vi "espectroscopia.vi"() -> ()   [LabVIEW 2016]
uses:
  indicador.ctl
  <vilib>/Utility/file.llb/Write Delimited Spreadsheet (DBL).vi
panel:
  in  "Ref. Mult":dbl
  in  "Ref. LockIn":dbl
  in  "movil":enum16{"acton", "spex"}(ring)
  in  "fijo":enum16{"acton", "spex"}(ring)
  out "medicion":T1
  in  "tipo":bool
  in  "OK Button":bool
  in  "Tab Control":enum32{"medir", "configurar"}(tab)
  out "Lamda Fija":dbl
  in  "Num.Lecturas":i32
  in  "Monocromador movil":cluster{"inicio":dbl, "fin":dbl, "paso":dbl}
  in  "Monocromador fijo":cluster{"Pos.":dbl}
  out "R 2":dbl
  out "DR 2":dbl
  out "DR/R 2":dbl
  out "Lamda":dbl
  in  "file path (use dialog)":path
  in  "spex":bool
  in  "acton":bool
  out "Long Acton":dbl
  in  "longitud Acton":dbl
  out "Longitud  de onda":dbl
  in  "longitud Spex":dbl
  in  "Detener":bool
  out "DR/R":cluster{dbl[], dbl[]}(graph)
  out "R":cluster{dbl[], dbl[]}(graph)
  out "DR":cluster{dbl[], dbl[]}(graph)
  # "PRE"
  # "PR"
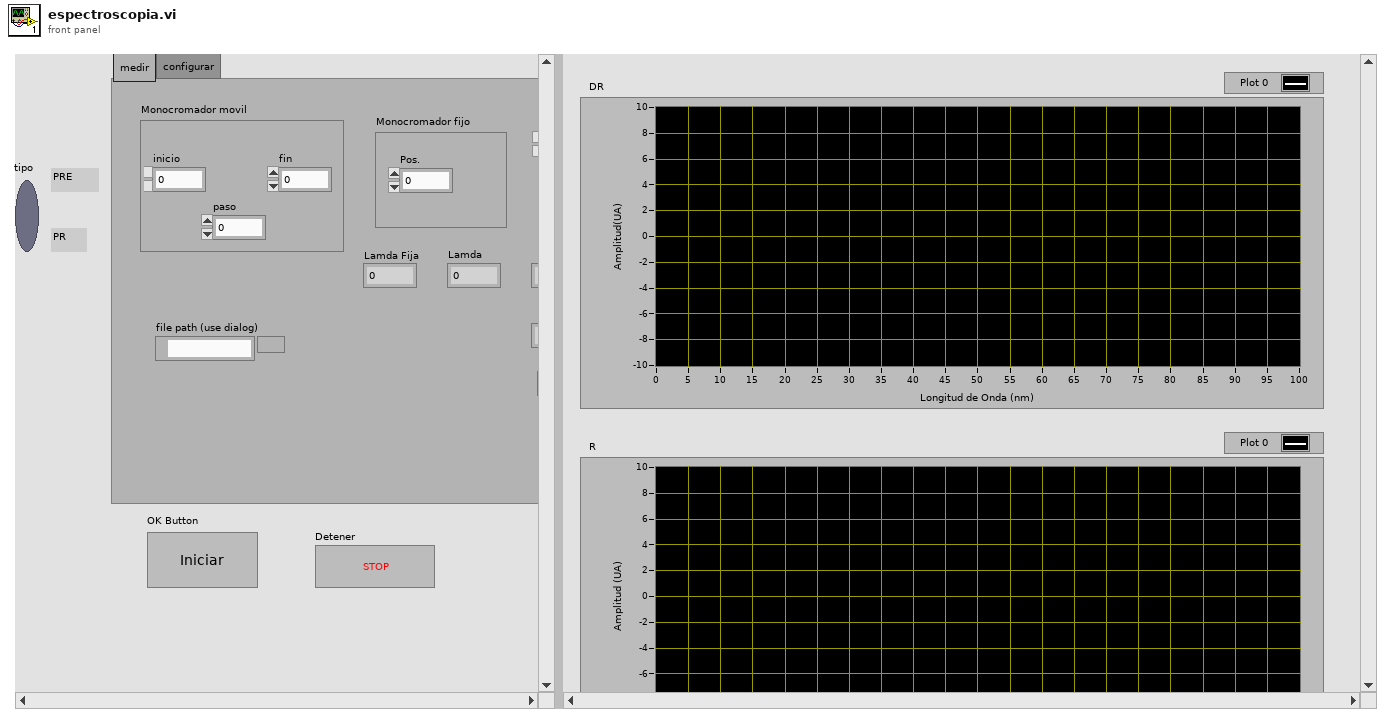
[diagram p1: front panel]
types:
  T1 = typedef "indicador.ctl" = bool
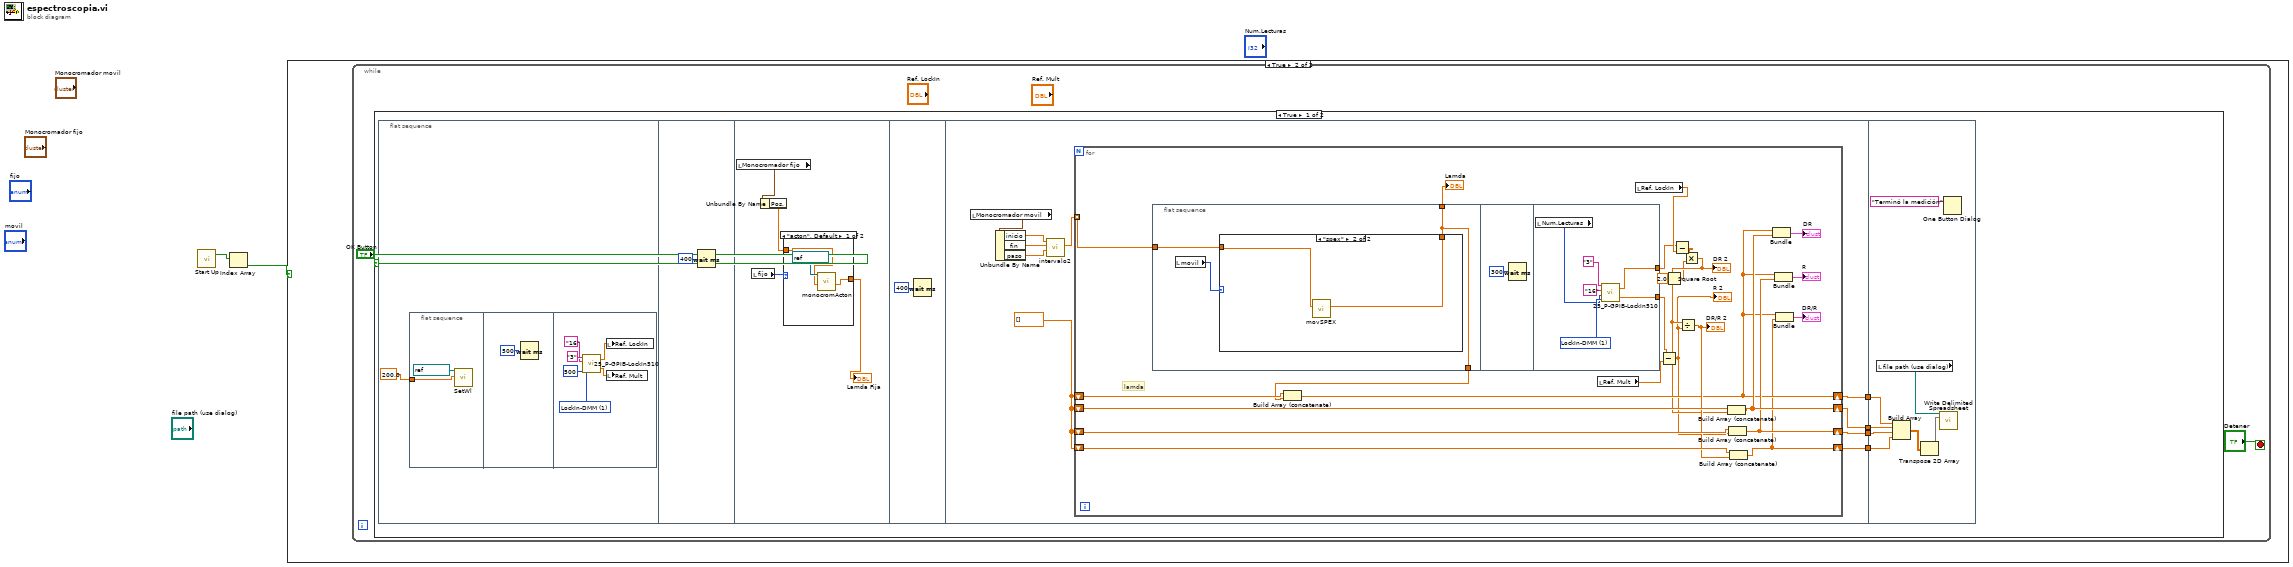
[diagram p0: block diagram]
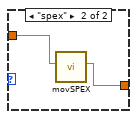
[diagram p3: hidden frame]
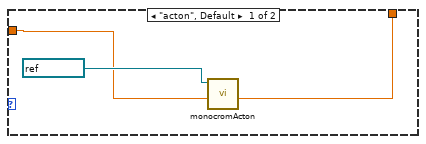
[diagram p4: hidden frame]
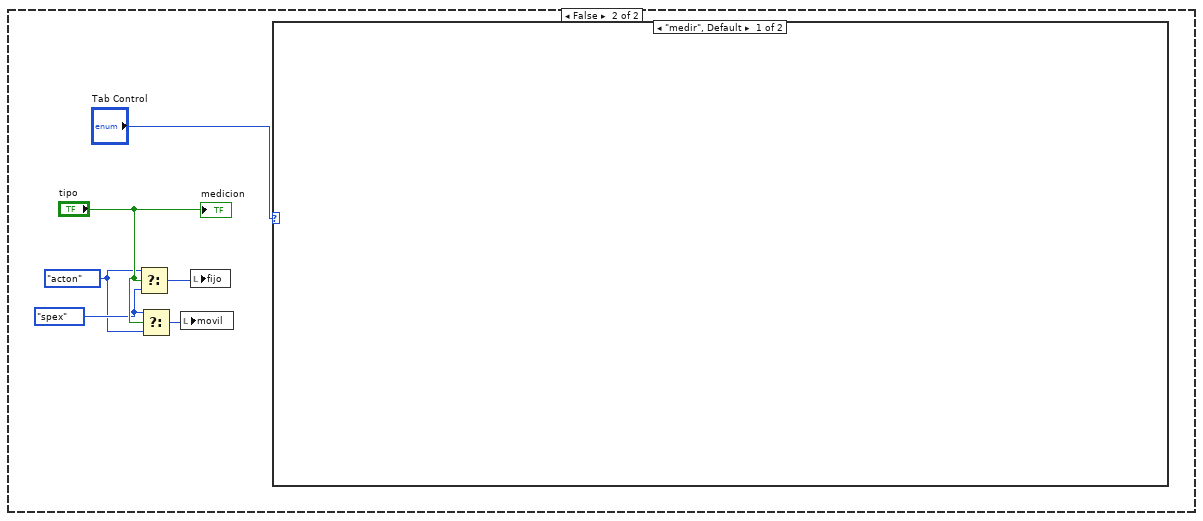
[diagram p5: hidden frame]
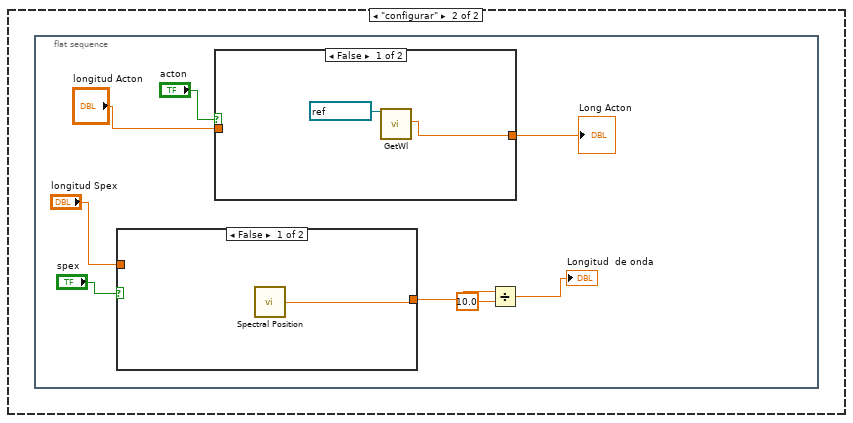
[diagram p6: hidden frame]
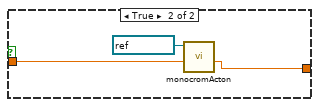
[diagram p7: hidden frame]
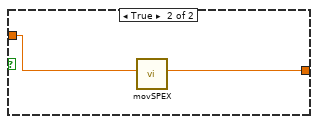
[diagram p8: hidden frame]
diagram:
  n1 = call "Start Up.VI"() -> ("Error List"=w2:bool[])  [unwired: 1 in, 1 out]
  n2 = Index Array(array=w2) -> (element=w1:bool)  [unwired: 1 in]
  n3 = case shown="True" w1 {
    frame False {
    }
    frame True {
      n4 = while {
        stop <- "Detener" stop-if-true
        n5 = case shown="True" "OK Button" {
          frame True {
            n6 = flat-sequence {
              tunnel: [w33] -> w8
              tunnel: [w32] -> w7
              tunnel: [w31] -> w6
              tunnel: [w30] -> w5
              tunnel: w8 -> [w84]
              tunnel: w7 -> [w83]
              tunnel: w6 -> [w82]
              tunnel: w5 -> [w81]
              frame #0 {
                n7 = flat-sequence {
                  tunnel: 200.0 -> [w10]
                  frame #0 {
                    n8 = call "SetWl.vi"("VISA resource name"=refnum<visa-resource-name> "COM5", "Wavelength (nm)"=w10) -> ()  [unwired: 16 in, 2 out]
                  }
                  frame #1 {
                    n9 = Wait (ms)(milliseconds to wait=u32 500) -> ()  [unwired: 1 out]
                  }
                  frame #2 {
                    w13 = u16 1 items=["LockIn", "LockIn-DMM"] ("Tipo")
                    n10 = call "25_P-GPIB-LockIn510.vi"("Tipo"=w13, "Lecturas"=500, "P-DMM"="16", "P-LockIn"="3") -> ("DMM"=w16:dbl, "LockIn"=w15:dbl)
                    n11 = local write "Ref. LockIn"(w15) -> ()
                    n12 = local write "Ref. Mult"(w16) -> ()
                  }
                }
              }
              frame #1 {
                n13 = Wait (ms)(milliseconds to wait=u32 400) -> ()  [unwired: 1 out]
              }
              frame #2 {
                n14 = local read "Monocromador fijo"() -> (w22:cluster{"Pos.":dbl})
                n15 = local read "fijo"() -> (w23:enum16{"acton", "spex"})
                n16 = Unbundle By Name(w22) -> ("Pos."=w21:dbl)
                n17 = case shown="\"acton\", Default" w23 {
                  tunnel: w21 -> [w25 w28]
                  tunnel: [w24 w27] -> w20
                  frame "acton", Default {
                    n18 = call "monocromActon.vi"("Lamda"=w25, "VISA resource name"=refnum<visa-resource-name> "COM3") -> ("Sal:Lamda"=w24:dbl)  [unwired: 9 in]
                  }
                  frame "spex" {
                    n19 = call "movSPEX.vi"("longitud de onda"=w28) -> ("Lamda"=w27:dbl)  [unwired: 10 in]
                  }
                }
                "Lamda Fija" <- w20
              }
              frame #3 {
                n20 = Wait (ms)(milliseconds to wait=u32 400) -> ()  [unwired: 1 out]
              }
              frame #4 {
                w34 = dbl[] []
                n21 = local read "Monocromador movil"() -> (w39:cluster{"inicio":dbl, "fin":dbl, "paso":dbl})
                n22 = Unbundle By Name(w39) -> ("inicio"=w38:dbl, "fin"=w37:dbl, "paso"=w36:dbl)
                n23 = call "intervalo2.vi"("incremento"=w36, "fin"=w37, "inicio"=w38) -> ("Array"=w35:dbl[])  [unwired: 8 in]
                n24 = for {
                  tunnel: w35 -> [w63] mode=indexing
                  shift-right: [w54] -> w32
                  shift-left: w34 -> [w59]
                  shift-right: [w52] -> w31
                  shift-left: w34 -> [w58]
                  shift-right: [w50] -> w30
                  shift-left: w34 -> [w57]
                  shift-right: [w51] -> w33
                  shift-left: w34 -> [w61]
                  # "lamda"
                  n25 = flat-sequence {
                    tunnel: w63 -> [w65]
                    tunnel: [w64] -> w62
                    tunnel: [w64] -> w60
                    tunnel: [w74] -> w45
                    tunnel: [w73] -> w41
                    frame #0 {
                      n26 = local read "movil"() -> (w66:enum16{"acton", "spex"})
                      n27 = case shown="\"spex\"" w66 {
                        tunnel: w65 -> [w68 w71]
                        tunnel: [w67 w70] -> w64
                        frame "acton", Default {
                          n28 = call "monocromActon.vi"("Lamda"=w68, "VISA resource name"=refnum<visa-resource-name> "COM3") -> ("Sal:Lamda"=w67:dbl)  [unwired: 9 in]
                        }
                        frame "spex" {
                          n29 = call "movSPEX.vi"("longitud de onda"=w71) -> ("Lamda"=w70:dbl)  [unwired: 10 in]
                        }
                      }
                    }
                    frame #1 {
                      n30 = Wait (ms)(milliseconds to wait=u32 300) -> ()  [unwired: 1 out]
                    }
                    frame #2 {
                      w76 = u16 1 items=["LockIn", "LockIn-DMM"] ("Tipo")
                      n31 = local read "Num.Lecturas"() -> (w75:i32)
                      n32 = call "25_P-GPIB-LockIn510.vi"("Tipo"=w76, "Lecturas"=w75, "P-DMM"="16", "P-LockIn"="3") -> ("DMM"=w73:dbl, "LockIn"=w74:dbl)
                    }
                  }
                  n33 = Build Array (concatenate)(w61, w60) -> (w51:dbl[])
                  n34 = local read "Ref. Mult"() -> (w40:dbl)
                  n35 = local read "Ref. LockIn"() -> (w48:dbl)
                  n36 = Subtract(x=w41, y=w40) -> (x-y=w42:dbl)
                  "R 2" <- w42
                  n37 = Square Root(x=2.0) -> (sqrt(x)=w44:dbl)
                  n38 = Subtract(x=w45, y=w48) -> (x-y=w47:dbl)
                  n39 = Multiply(x=w47, y=w44) -> (x*y=w46:dbl)
                  "DR 2" <- w46
                  n40 = Divide(x=w46, y=w42) -> (x/y=w56:dbl)
                  "DR/R 2" <- w56
                  n41 = Build Array (concatenate)(w59, w46) -> (w54:dbl[])
                  n42 = Build Array (concatenate)(w58, w42) -> (w52:dbl[])
                  n43 = Build Array (concatenate)(w57, w56) -> (w50:dbl[])
                  n44 = Bundle(w51, w54) -> (→"DR":cluster{dbl[], dbl[]})  [unwired: 1 in]
                  n45 = Bundle(w51, w52) -> (→"R":cluster{dbl[], dbl[]})  [unwired: 1 in]
                  n46 = Bundle(w51, w50) -> (→"DR/R":cluster{dbl[], dbl[]})  [unwired: 1 in]
                  "Lamda" <- w62
                }
              }
              frame #5 {
                n47 = local read "file path (use dialog)"() -> (w85:path)
                n48 = Build Array(w84, w83, w82, w81) -> (w80:dbl[][])
                n49 = Transpose 2D Array(2D array=w80) -> (transposed array=w79:dbl[][])
                n50 = call-poly <vilib>:"Write Delimited Spreadsheet.vi"("file path (dialog if empty)"=w85, "2D data"=w79) -> ()  [unwired: 12 in, 2 out]
                n51 = One Button Dialog(message="Terminó la medición") -> ()  [unwired: 1 in, 1 out]
              }
            }
          }
          frame False {
            w89 = enum16{"acton", "spex"}."spex" ("fijo")
            w88 = enum16{"acton", "spex"}."acton" ("fijo")
            n52 = Select(t=w88, s="tipo", f=w89) -> (s? t:f=w91:enum16{"acton", "spex"})
            n53 = Select(t=w89, s="tipo", f=w88) -> (s? t:f=w87:enum16{"acton", "spex"})
            n54 = local write "movil"(w87) -> ()
            n55 = local write "fijo"(w91) -> ()
            n56 = case shown="\"medir\", Default" "Tab Control" {
              frame "medir", Default {
              }
              frame "configurar" {
                n57 = flat-sequence {
                  frame #0 {
                    n58 = case shown="False" "spex" {
                      tunnel: "longitud Spex" -> [_ w108]
                      tunnel: [w106 w107] -> w96
                      frame False {
                        n59 = call "Spectral Position.VI"() -> ("Present Position"=w106:dbl)  [unwired: 1 in, 2 out]
                      }
                      frame True {
                        n60 = call "movSPEX.vi"("longitud de onda"=w108) -> ("Lamda"=w107:dbl)  [unwired: 10 in]
                      }
                    }
                    n61 = case shown="False" "acton" {
                      tunnel: [w102 w105] -> w98
                      tunnel: "longitud Acton" -> [_ w104]
                      frame False {
                        n62 = call "GetWl.vi"("VISA resource name"=refnum<visa-resource-name> "COM3") -> ("Wavelength"=w102:dbl)  [unwired: 16 in, 2 out]
                      }
                      frame True {
                        n63 = call "monocromActon.vi"("Lamda"=w104, "VISA resource name"=refnum<visa-resource-name> "COM3") -> ("Sal:Lamda"=w105:dbl)  [unwired: 9 in]
                      }
                    }
                    "Long Acton" <- w98
                    n64 = Divide(x=w96, y=10.0) -> (x/y=→"Longitud  de onda":dbl)
                  }
                }
              }
            }
            "medicion" <- "tipo"
          }
        }
      }
    }
  }
